vi "Add Update Node.vi"(8 "error in (no error)":errorcluster, 10 "Test Event":T1, 11 "Test Event Storage in":refnum<class "Test Event Storage.lvclass">) -> (0 "error out":errorcluster, 1 "Key":string, 2 "found?":bool, 3 "Test Event Storage out":refnum<class "Test Event Storage.lvclass">)   [LabVIEW 2009, in "Caraya.lvlib" / "Test Event Storage.lvclass"]
uses:
  Test Event Storage.lvclass
  Basic Test Manager/Assert Event Data.ctl
  Test Node.ctl
  Basic Test Manager/Test Registration Data.ctl
  Test Event Storage.lvclass/Test Event Storage.ctl
  Basic Test Manager/Basic Test Manager.lvclass
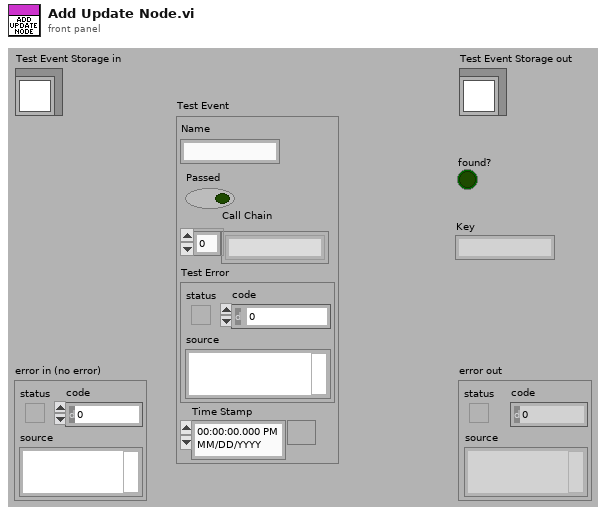
[diagram p1: front panel]
types:
  T1 = typedef "Caraya.lvlib/Basic Test Manager.lvclass/Assert Event Data.ctl" = cluster{"Name":string, "Passed":bool, "Call Chain":string[], "Test Error":errorcluster, "Time Stamp":timestamp}
  T2 = typedef "Caraya.lvlib/Test Event Storage.lvclass/Test Node.ctl" = cluster{"Test Registration":T3, "Defined":bool, "Passed":bool}
  T3 = typedef "Caraya.lvlib/Basic Test Manager.lvclass/Test Registration Data.ctl" = cluster{"Name":string, "Call Chain":string[], "Time Stamp":timestamp}
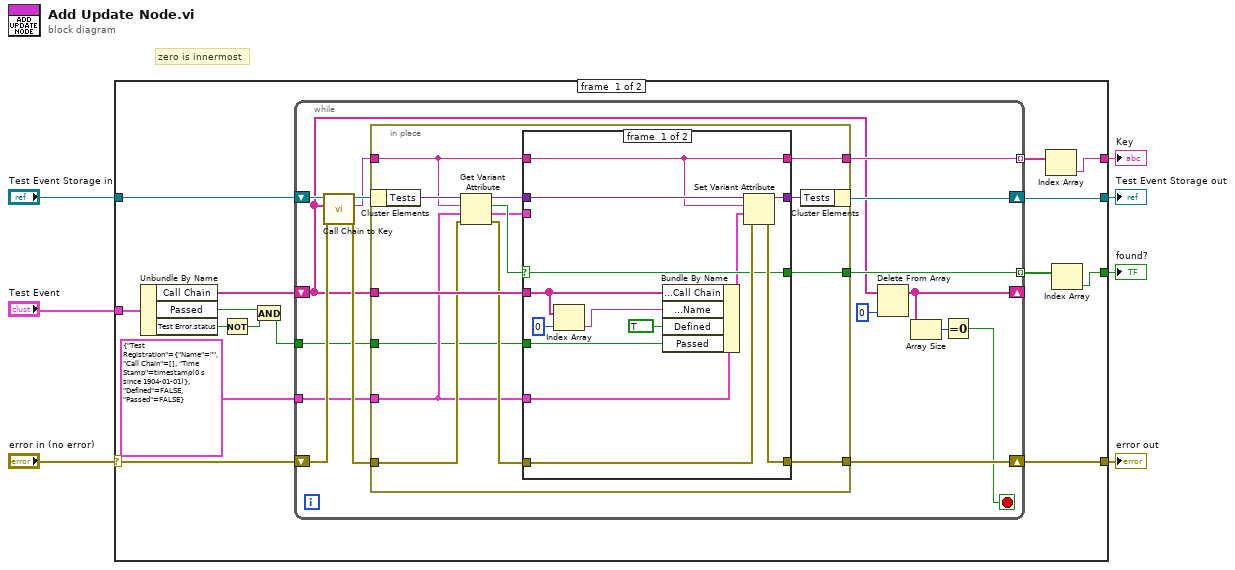
[diagram p0: block diagram]
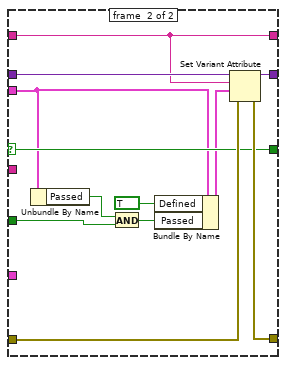
[diagram p2: hidden frame]
diagram:
  # "zero is innermost"
  n1 = case shown="No Error" "error in (no error)" {
    selector: "error in (no error)" -> [w21 w79]
    tunnel: [w20 w79] -> w6
    tunnel: [w19 w78] -> w4
    tunnel: "Test Event Storage in" -> [w22 w78]
    tunnel: [w8 _] -> w3
    tunnel: "Test Event" -> [w18 _]
    tunnel: [w10 _] -> w1
    frame #0 {
      n2 = Unbundle By Name(w18) -> ("Call Chain"=w17:string[], "Passed"=w15:bool, "Test Error.status"=w13:bool)
      n3 = Not(x=w13) -> (.not. x?=w14:bool)
      n4 = And(x=w15, y=w14) -> (x .and. y?=w12:bool)
      n5 = while {
        tunnel: [w31] -> w9 mode=indexing
        tunnel: [w30] -> w11 mode=indexing
        tunnel: T2 {"Test Registration"={"Name"="", "Call Chain"=[], "Time Stamp"=timestamp(0 s since 1904-01-01)}, "Defined"=FALSE, "Passed"=FALSE} ("Test Node") -> [w29]
        tunnel: w12 -> [w28]
        shift-right: [w25] -> _
        shift-left: w17 -> [w27]
        shift-right: [w32] -> w19
        shift-left: w22 -> [w38]
        shift-right: [w33] -> w20
        shift-left: w21 -> [w36]
        stop <- w23 stop-if-true
        n6 = call "Call Chain to Key.vi"("error in (no error)"=w36, "Call Chain"=w27, "Test Event Storage in"=w38) -> ("error out"=w35:errorcluster, "Key"=w34:string, "Test Event Storage out"=w37:refnum<class "Test Event Storage.lvclass">)  [unwired: 6 in]
        n7 = in-place {
          in-place-border: w35 -> [w45]
          in-place-border: w34 -> [w47]
          in-place-border: w27 -> [w50]
          in-place-border: [w51] -> w33
          in-place-border: [w49] -> w31
          in-place-border: w29 -> [w42]
          in-place-border: [w41] -> w30
          in-place-border: w28 -> [w40]
          n8 = in-place-cluster #1(w37) -> ("Tests"=w48:variant)
          n9 = Get Variant Attribute(Variant=w48, name=w47, default value (empty Variant)=w42, error in=w45) -> (duplicate Variant=w46:variant, found=w43:bool, value=w39:T2, error out=w44:errorcluster)
          n10 = case shown="False" w43 {
            selector: w43 -> [w61 w73]
            tunnel: [w65 w77] -> w52
            tunnel: [w64 w76] -> w51
            tunnel: w50 -> [w57 _]
            tunnel: [w61 w73] -> w49
            tunnel: w47 -> [w58 w71]
            tunnel: w46 -> [w63 w75]
            tunnel: w44 -> [w62 w74]
            tunnel: w42 -> [w60 _]
            tunnel: [w58 w71] -> w41
            tunnel: w40 -> [w54 w66]
            tunnel: w39 -> [_ w70]
            frame #0 {
              n11 = Index Array(array=w57, index=0) -> (element=w55:string)
              n12 = Bundle By Name(cluster=w60, "Test Registration.Call Chain"=w57, "Test Registration.Name"=w55, "Defined"=TRUE, "Passed"=w54) -> (w59:T2)
              n13 = Set Variant Attribute(Variant=w63, name=w58, value=w59, error in=w62) -> (Variant out=w65:variant, error out=w64:errorcluster)  [unwired: 1 out]
            }
            frame #1 {
              n14 = Unbundle By Name(w70) -> ("Passed"=w68:bool)
              n15 = And(x=w68, y=w66) -> (x .and. y?=w67:bool)
              n16 = Bundle By Name(cluster=w70, "Defined"=TRUE, "Passed"=w67) -> (w72:T2)
              n17 = Set Variant Attribute(Variant=w75, name=w71, value=w72, error in=w74) -> (Variant out=w77:variant, error out=w76:errorcluster)  [unwired: 1 out]
            }
          }
          n18 = in-place-cluster #1("Tests"=w52) -> (w32:refnum<class "Test Event Storage.lvclass">)
        }
        n19 = Delete From Array(array=w27, index=0) -> (array with subset deleted=w25:string[])  [unwired: 1 in, 1 out]
        n20 = Array Size(array=w25) -> (size(s)=w24:i32)
        n21 = Equal To 0?(x=w24) -> (x = 0?=w23:bool)
      }
      n22 = Index Array(array=w11) -> (element=w10:string)  [unwired: 1 in]
      n23 = Index Array(array=w9) -> (element=w8:bool)  [unwired: 1 in]
    }
    frame #1 {
    }
  }
  "error out" <- w6
  "Test Event Storage out" <- w4
  "found?" <- w3
  "Key" <- w1
